vi "Day 20-Add Padding2.vi"(10 "Padding Value":bool, 11 "Array in":bool[][](array[boolean])) -> (3 "Array out":bool[][](array[boolean]))   [LabVIEW 2021]
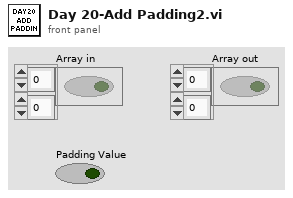
[diagram p1: front panel]
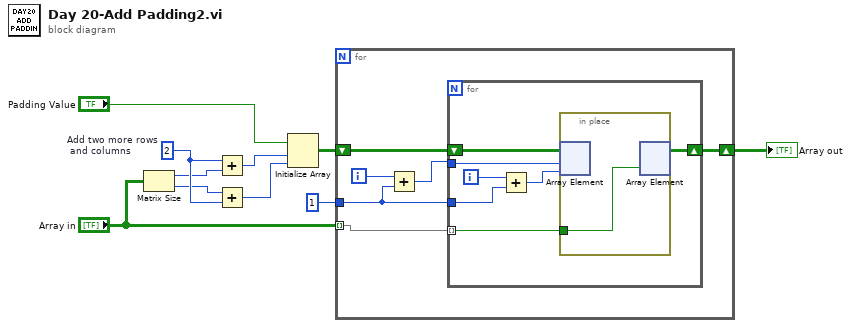
[diagram p0: block diagram]
diagram:
  w7 = 2  # Add two more rows  and columns
  n1 = Matrix Size(0:"Array in") -> (1:w4:i32, 2:w3:i32)
  n2 = Add(x=w7, y=w4) -> (x+y=w1:i32)
  n3 = Add(x=w3, y=w7) -> (x+y=w2:i32)
  n4 = Initialize Array("Padding Value", w1, w2) -> (w5:bool[][])
  n5 = for {
    tunnel: "Array in" -> [w15] mode=indexing
    shift-right: [w14] -> w9
    shift-left: w5 -> [w16]
    tunnel: 1 -> [w11]
    i -> [w13]
    n6 = Add(x=w13, y=w11) -> (x+y=w12:i32)
    n7 = for {
      shift-right: [w20] -> w14
      shift-left: w16 -> [w23]
      tunnel: w12 -> [w22]
      tunnel: w15 -> [w21] mode=indexing
      tunnel: w11 -> [w17]
      i -> [w19]
      n8 = Add(x=w19, y=w17) -> (x+y=w18:i32)
      n9 = in-place {
        in-place-border: w21 -> [w24]
        n10 = in-place-array #1(w23, w22, w18) -> ()  [unwired: 1 out]
        n11 = in-place-array #1(w24) -> (w20:bool[][])  [unwired: 2 out]
      }
    }
  }
  "Array out" <- w9
